vi "Get Broken VIs.vi"(8 "error in (no error)":errorcluster, 11 "NI_AB_API_Build in":refnum<class "NI_AB_API_Build.lvclass">) -> (0 "error out":errorcluster, 1 "before build?":bool, 2 "Broken VI List":string[](array[string]), 3 "NI_AB_API_Build out":refnum<class "NI_AB_API_Build.lvclass">, 5 "Has errors?":bool=TRUE)   [LabVIEW 2020, in "NI_AB_API_Build.lvclass"]
uses:
  <vilib>/AppBuilder/AB_API/Build/NI_AB_API_Build.lvclass
  <vilib>/AppBuilder/AB_API/Build/NI_AB_API_Build.lvclass/NI_AB_API_Build.ctl
  <vilib>/AppBuilder/AB_Classes/Build/AB_Build.lvclass
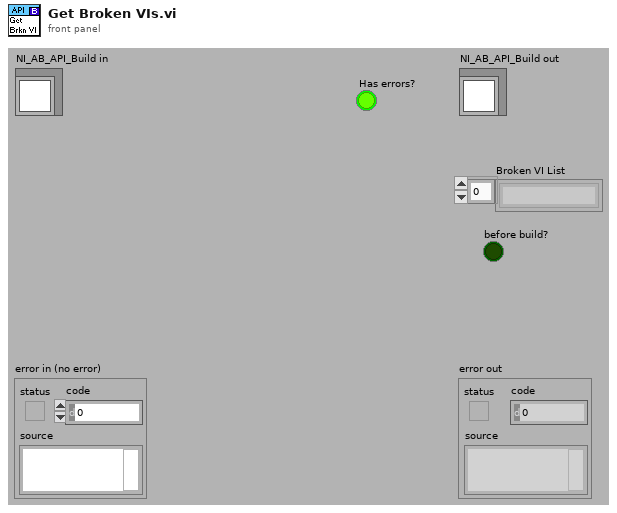
[diagram p1: front panel]
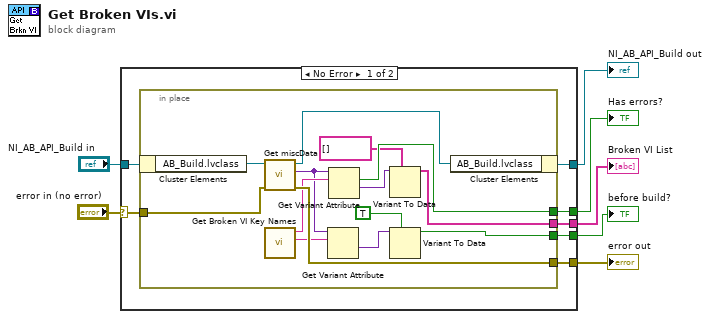
[diagram p0: block diagram]
diagram:
  n1 = case shown="No Error" "error in (no error)" {
    selector: "error in (no error)" -> [w11 w30]
    tunnel: [w10 w30] -> w6
    tunnel: [w8 w29] -> w4
    tunnel: "NI_AB_API_Build in" -> [w9 w29]
    tunnel: [w14 _] -> w3
    tunnel: [w13 _] -> w2
    tunnel: [w12 _] -> w1
    frame No Error {
      n2 = in-place {
        in-place-border: [w28] -> w14
        in-place-border: [w27] -> w13
        in-place-border: [w26] -> w12
        in-place-border: w11 -> [w25]
        in-place-border: [w24] -> w10
        n3 = in-place-cluster #1(w9) -> ("AB_Build.lvclass"=w16:refnum<class "AB_Build.lvclass">)
        n4 = call-dynamic "Get miscData.vi"("error in (no error)"=w25, "AB_Build in"=w16) -> ("error out"=w24:errorcluster, "eng_miscData"=w20:variant, "AB_Build out"=w15:refnum<class "AB_Build.lvclass">)  [unwired: 7 in]
        n5 = call <vilib>:"Get Broken VI Key Names.vi"() -> ("Before Build Key"=w19:string, "Broken VIs List Key"=w23:string)  [unwired: 10 in]
        n6 = Get Variant Attribute(Variant=w20, name=w19) -> (value=w17:variant)  [unwired: 2 in, 3 out]
        n7 = Get Variant Attribute(Variant=w20, name=w23) -> (found=w27:bool, value=w22:variant)  [unwired: 2 in, 2 out]
        n8 = Variant To Data(type=string[] [] ("Broken VI List"), Variant=w22) -> (data=w28:string[])  [unwired: 1 in, 1 out]
        n9 = Variant To Data(type=TRUE ("Has errors?"), Variant=w17) -> (data=w26:bool)  [unwired: 1 in, 1 out]
        n10 = in-place-cluster #1("AB_Build.lvclass"=w15) -> (w8:refnum<class "NI_AB_API_Build.lvclass">)
      }
    }
    frame Error {
    }
  }
  "error out" <- w6
  "NI_AB_API_Build out" <- w4
  "Has errors?" <- w2
  "Broken VI List" <- w3
  "before build?" <- w1
